vi "9220 16Ch Analog Input.vi"(1 "9220 I/O":T1={"9220 AI0"="NI 9220/AI0", "9220 AI1"="NI 9220/AI1", "9220 AI2"="NI 9220/AI2", "9220 AI3"="NI 9220/AI3", "9220 AI4"="NI 9220/AI4", "9220 AI5"="NI 9220/AI5", "9220 AI6"="NI 9220/AI6", "9220 AI7"="NI 9220/AI7", "9220 AI8"="NI 9220/AI8", "9220 AI9"="NI 9220/AI9", "9220 AI10"="NI 9220/AI10", "9220 AI11"="NI 9220/AI11", "9220 AI12"="NI 9220/AI12", "9220 AI13"="NI 9220/AI13", "9220 AI14"="NI 9220/AI14", "9220 AI15"="NI 9220/AI15"}) -> (0 "Packets":u64[](array[numeric]))   [LabVIEW 2010]
uses:
  <vilib>/eio/EIONode/EIONode.xnode
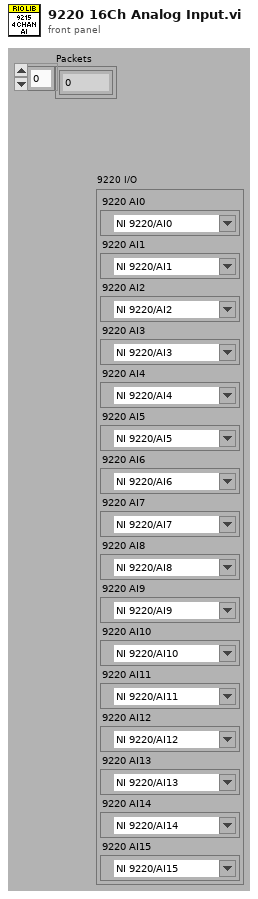
[diagram p1: front panel]
types:
  T1 = cluster{"9220 AI0":refnum<k21>, "9220 AI1":refnum<k21>, "9220 AI2":refnum<k21>, "9220 AI3":refnum<k21>, "9220 AI4":refnum<k21>, "9220 AI5":refnum<k21>, "9220 AI6":refnum<k21>, "9220 AI7":refnum<k21>, "9220 AI8":refnum<k21>, "9220 AI9":refnum<k21>, "9220 AI10":refnum<k21>, "9220 AI11":refnum<k21>, "9220 AI12":refnum<k21>, "9220 AI13":refnum<k21>, "9220 AI14":refnum<k21>, "9220 AI15":refnum<k21>}
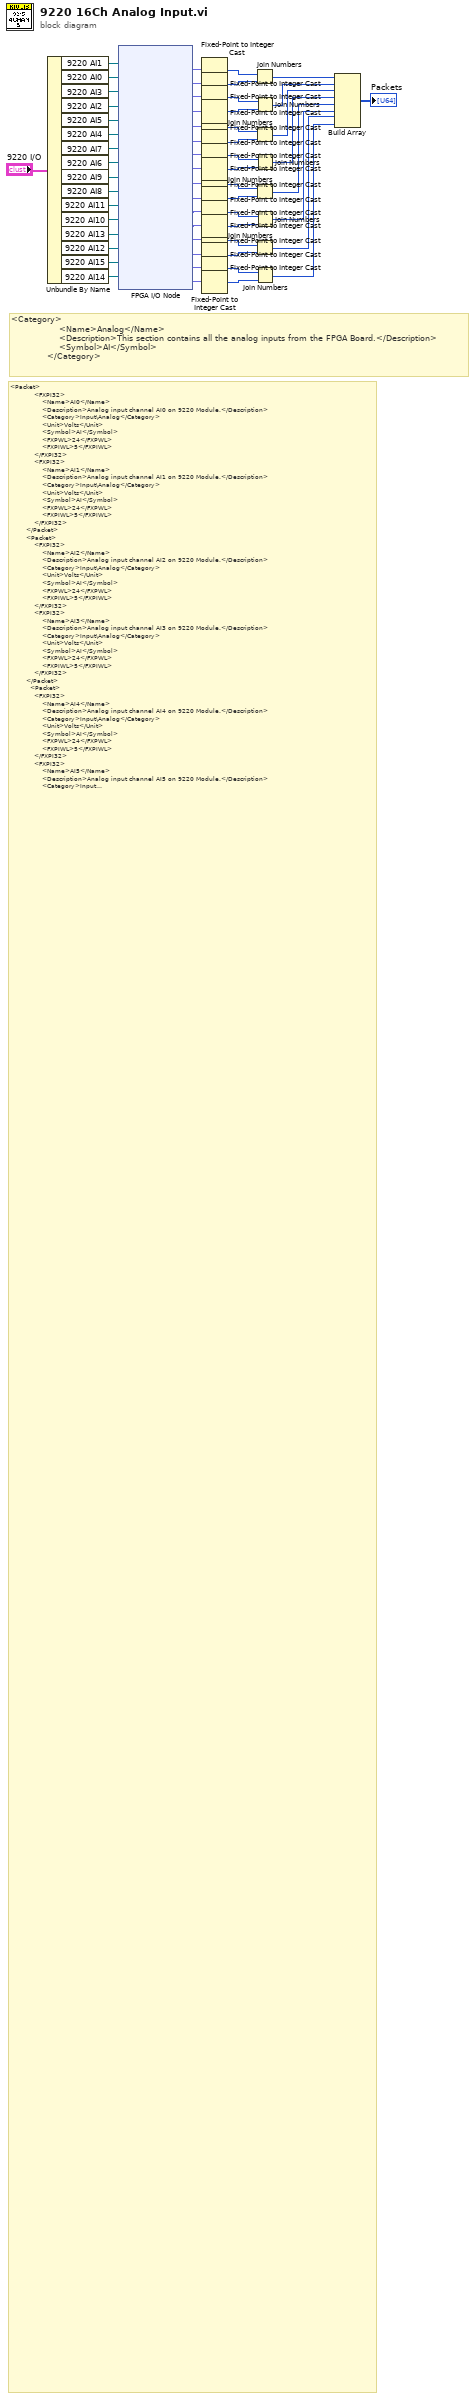
[diagram p0: block diagram]
diagram:
  # "<Category>\n                <Name>Analog</Name>\n                <Description>This section contains all the analog inputs from the FPGA Board.</Description>\n                <Symbol>AI</Symbol>\n            </Category>"
  # "<Packet>\n            <FXPI32>\n                <Name>AI0</Name>\n                <Description>Analog input channel AI0 on 9220 Module.</Description>\n                <Category>Input\\Analog</Category>\n                <Unit>Volts</Unit>\n                <Symbol>AI</Symbol>\n                <FXPWL>24</FXPWL>\n                <FXPIWL>5</FXPIWL>\n            </FXPI32>\n            <FXPI32>\n                <Name>AI1</Name>\n                <Description>Analog input channel AI1 on 9220 Module.</Description>\n                <Category>Input\\Analog</Category>\n                <Unit>Volts</Unit>\n                <Symbol>AI</Symbol>\n                <FXPWL>24</FXPWL>\n                <FXPIWL>5</FXPIWL>\n            </FXPI32>\n        </Packet>\n        <Packet>\n            <FXPI32>\n                <Name>AI2</Name>\n                <Description>Analog input channel AI2 on 9220 Module.</Description>\n                <Category>Input\\Analog</Category>\n                <Unit>Volts</Unit>\n                <Symbol>AI</Symbol>\n                <FXPWL>24</FXPWL>\n                <FXPIWL>5</FXPIWL>\n            </FXPI32>\n            <FXPI32>\n                <Name>AI3</Name>\n                <Description>Analog input channel AI3 on 9220 Module.</Description>\n                <Category>Input\\Analog</Category>\n                <Unit>Volts</Unit>\n                <Symbol>AI</Symbol>\n                <FXPWL>24</FXPWL>\n                <FXPIWL>5</FXPIWL>\n            </FXPI32>\n        </Packet>\n\t\t        <Packet>\n            <FXPI32>\n                <Name>AI4</Name>\n                <Description>Analog input channel AI4 on 9220 Module.</Description>\n                <Category>Input\\Analog</Category>\n                <Unit>Volts</Unit>\n                <Symbol>AI</Symbol>\n                <FXPWL>24</FXPWL>\n                <FXPIWL>5</FXPIWL>\n            </FXPI32>\n            <FXPI32>\n                <Name>AI5</Name>\n                <Description>Analog input channel AI5 on 9220 Module.</Description>\n                <Category>Input\\Analog</Category>\n                <Unit>Volts</Unit>\n                <Symbol>AI</Symbol>\n                <FXPWL>24</FXPWL>\n                <FXPIWL>5</FXPIWL>\n            </FXPI32>\n        </Packet>\n        <Packet>\n            <FXPI32>\n                <Name>AI6</Name>\n                <Description>Analog input channel AI6 on 9220 Module.</Description>\n                <Category>Input\\Analog</Category>\n                <Unit>Volts</Unit>\n                <Symbol>AI</Symbol>\n                <FXPWL>24</FXPWL>\n                <FXPIWL>5</FXPIWL>\n            </FXPI32>\n            <FXPI32>\n                <Name>AI7</Name>\n                <Description>Analog input channel AI7 on 9220 Module.</Description>\n                <Category>Input\\Analog</Category>\n                <Unit>Volts</Unit>\n                <Symbol>AI</Symbol>\n                <FXPWL>24</FXPWL>\n                <FXPIWL>5</FXPIWL>\n            </FXPI32>\n        </Packet>\n\t\t        <Packet>\n            <FXPI32>\n                <Name>AI8</Name>\n                <Description>Analog input channel AI8 on 9220 Module.</Description>\n                <Category>Input\\Analog</Category>\n                <Unit>Volts</Unit>\n                <Symbol>AI</Symbol>\n                <FXPWL>24</FXPWL>\n                <FXPIWL>5</FXPIWL>\n            </FXPI32>\n            <FXPI32>\n                <Name>AI9</Name>\n                <Description>Analog input channel AI9 on 9220 Module.</Description>\n                <Category>Input\\Analog</Category>\n                <Unit>Volts</Unit>\n                <Symbol>AI</Symbol>\n                <FXPWL>24</FXPWL>\n                <FXPIWL>5</FXPIWL>\n            </FXPI32>\n        </Packet>\n        <Packet>\n            <FXPI32>\n                <Name>AI10</Name>\n                <Description>Analog input channel AI10 on 9220 Module.</Description>\n                <Category>Input\\Analog</Category>\n                <Unit>Volts</Unit>\n                <Symbol>AI</Symbol>\n                <FXPWL>24</FXPWL>\n                <FXPIWL>5</FXPIWL>\n            </FXPI32>\n            <FXPI32>\n                <Name>AI11</Name>\n                <Description>Analog input channel AI11 on 9220 Module.</Description>\n                <Category>Input\\Analog</Category>\n                <Unit>Volts</Unit>\n                <Symbol>AI</Symbol>\n                <FXPWL>24</FXPWL>\n                <FXPIWL>5</FXPIWL>\n            </FXPI32>\n        </Packet>\n\t\t        <Packet>\n            <FXPI32>\n                <Name>AI12</Name>\n                <Description>Analog input channel AI12 on 9220 Module.</Description>\n                <Category>Input\\Analog</Category>\n                <Unit>Volts</Unit>\n                <Symbol>AI</Symbol>\n                <FXPWL>24</FXPWL>\n                <FXPIWL>5</FXPIWL>\n            </FXPI32>\n            <FXPI32>\n                <Name>AI13</Name>\n                <Description>Analog input channel AI13 on 9220 Module.</Description>\n                <Category>Input\\Analog</Category>\n                <Unit>Volts</Unit>\n                <Symbol>AI</Symbol>\n                <FXPWL>24</FXPWL>\n                <FXPIWL>5</FXPIWL>\n            </FXPI32>\n        </Packet>\n        <Packet>\n            <FXPI32>\n                <Name>AI14</Name>\n                <Description>Analog input channel AI14 on 9220 Module.</Description>\n                <Category>Input\\Analog</Category>\n                <Unit>Volts</Unit>\n                <Symbol>AI</Symbol>\n                <FXPWL>24</FXPWL>\n                <FXPIWL>5</FXPIWL>\n            </FXPI32>\n            <FXPI32>\n                <Name>AI15</Name>\n                <Description>Analog input channel AI15 on 9220 Module.</Description>\n                <Category>Input\\Analog</Category>\n                <Unit>Volts</Unit>\n                <Symbol>AI</Symbol>\n                <FXPWL>24</FXPWL>\n                <FXPIWL>5</FXPIWL>\n            </FXPI32>\n        </Packet>"
  n1 = Unbundle By Name("9220 I/O") -> ("9220 AI1"=w48:refnum<k21>, "9220 AI0"=w51:refnum<k21>, "9220 AI3"=w49:refnum<k21>, "9220 AI2"=w52:refnum<k21>, "9220 AI5"=w43:refnum<k21>, "9220 AI4"=w42:refnum<k21>, "9220 AI7"=w41:refnum<k21>, "9220 AI6"=w40:refnum<k21>, "9220 AI9"=w39:refnum<k21>, "9220 AI8"=w38:refnum<k21>, "9220 AI11"=w37:refnum<k21>, "9220 AI10"=w36:refnum<k21>, "9220 AI13"=w35:refnum<k21>, "9220 AI12"=w34:refnum<k21>, "9220 AI15"=w33:refnum<k21>, "9220 AI14"=w32:refnum<k21>)
  n2 = xnode "FPGA I/O Node"("FPGA I/O In"=w48, "FPGA I/O In"=w51, "FPGA I/O In"=w49, "FPGA I/O In"=w52, "FPGA I/O In"=w43, "FPGA I/O In"=w42, "FPGA I/O In"=w41, "FPGA I/O In"=w40, "FPGA I/O In"=w39, "FPGA I/O In"=w38, "FPGA I/O In"=w37, "FPGA I/O In"=w36, "FPGA I/O In"=w35, "FPGA I/O In"=w34, "FPGA I/O In"=w33, "FPGA I/O In"=w32) -> ("I/O Item"=w54:fxp<+/-,24,5>, "I/O Item"=w56:fxp<+/-,24,5>, "I/O Item"=w50:fxp<+/-,24,5>, "I/O Item"=w55:fxp<+/-,24,5>, "I/O Item"=w27:fxp<+/-,24,5>, "I/O Item"=w17:fxp<+/-,24,5>, "I/O Item"=w16:fxp<+/-,24,5>, "I/O Item"=w15:fxp<+/-,24,5>, "I/O Item"=w14:fxp<+/-,24,5>, "I/O Item"=w13:fxp<+/-,24,5>, "I/O Item"=w12:fxp<+/-,24,5>, "I/O Item"=w11:fxp<+/-,24,5>, "I/O Item"=w18:fxp<+/-,24,5>, "I/O Item"=w10:fxp<+/-,24,5>, "I/O Item"=w9:fxp<+/-,24,5>, "I/O Item"=w8:fxp<+/-,24,5>)  [unwired: 16 out]
  n3 = Fixed-Point to Integer Cast(1:w54) -> (0:w47:i32)
  n4 = Fixed-Point to Integer Cast(1:w56) -> (0:w46:i32)
  n5 = Fixed-Point to Integer Cast(1:w50) -> (0:w45:i32)
  n6 = Fixed-Point to Integer Cast(1:w55) -> (0:w44:i32)
  n7 = Fixed-Point to Integer Cast(1:w27) -> (0:w28:i32)
  n8 = Fixed-Point to Integer Cast(1:w17) -> (0:w29:i32)
  n9 = Fixed-Point to Integer Cast(1:w16) -> (0:w30:i32)
  n10 = Fixed-Point to Integer Cast(1:w15) -> (0:w31:i32)
  n11 = Fixed-Point to Integer Cast(1:w14) -> (0:w26:i32)
  n12 = Fixed-Point to Integer Cast(1:w13) -> (0:w25:i32)
  n13 = Fixed-Point to Integer Cast(1:w12) -> (0:w24:i32)
  n14 = Fixed-Point to Integer Cast(1:w11) -> (0:w23:i32)
  n15 = Fixed-Point to Integer Cast(1:w18) -> (0:w19:i32)
  n16 = Fixed-Point to Integer Cast(1:w10) -> (0:w20:i32)
  n17 = Fixed-Point to Integer Cast(1:w9) -> (0:w21:i32)
  n18 = Fixed-Point to Integer Cast(1:w8) -> (0:w22:i32)
  n19 = Join Numbers(hi=w47, lo=w46) -> ((hi.lo)=w57:u64)
  n20 = Join Numbers(hi=w28, lo=w29) -> ((hi.lo)=w7:u64)
  n21 = Join Numbers(hi=w26, lo=w25) -> ((hi.lo)=w5:u64)
  n22 = Join Numbers(hi=w19, lo=w20) -> ((hi.lo)=w3:u64)
  n23 = Join Numbers(hi=w45, lo=w44) -> ((hi.lo)=w58:u64)
  n24 = Join Numbers(hi=w30, lo=w31) -> ((hi.lo)=w6:u64)
  n25 = Join Numbers(hi=w24, lo=w23) -> ((hi.lo)=w4:u64)
  n26 = Join Numbers(hi=w21, lo=w22) -> ((hi.lo)=w2:u64)
  n27 = Build Array(w57, w58, w7, w6, w5, w4, w3, w2) -> (→"Packets":u64[])
